vi "_SBR_mes_sp.vi"(6 "SBR_Set":T3={"file_name"="", "HOT/COLD AUTO"=TRUE, "MPI SSB Set"=TRUE, "AUTO時待ち時間（S）"=1.0, "P/V         V/P"=FALSE, "save"=TRUE, "start(GHz)"=4.0, "stop(GHz) "=12.0, "Step(GHz) "=0.1, "P.M.aveg"=10, "PM        SP"=FALSE, "SP_set"={"start(GHz)"=3.5, "stop(GHz) "=12.5, "BW(MHz)"=8.0, "VBW(Hz)"=30.0, "ref(dBm)"=-45.0, "log(dB)"=1.0, "AVEG"=1, "AVEG ON/OFF"=FALSE, "Auto Align ON/OFF"=FALSE, "GPIB"="18", "point"=801}}, 7 "Control":T2={"GPIB_ATT"="28", "6501Dev#"=1, "GPIB_SP"="18", "GPIB_PM"="13", "GPIB_DSA"="11", "GPIB_DMM (TPD)"="23", "MPICOM"="COM5", "mortor設定"=[{"Axis"=0, "ID"=0, "HIspeed"=200.0, "LOspeed"=100.0, "ACCEL(ms)"=100.0, "Sratio"=50.0, "フリーラン\n"=FALSE, "文字列"="DSB HOT/COLD"}, {"Axis"=1, "ID"=0, "HIspeed"=4.0, "LOspeed"=4.0, "ACCEL(ms)"=100.0, "Sratio"=50.0, "フリーラン\n"=TRUE, "文字列"="SubMM Att"}, {"Axis"=0, "ID"=0, "HIspeed"=200.0, "LOspeed"=100.0, "ACCEL(ms)"=100.0, "Sratio"=50.0, "フリーラン\n"=FALSE, "文字列"="MPI Port1"}, {"Axis"=1, "ID"=0, "HIspeed"=200.0, "LOspeed"=100.0, "ACCEL(ms)"=100.0, "Sratio"=50.0, "フリーラン\n"=FALSE, "文字列"="MPI Port2"}], "DATAパス"=path "C:/Documents and Settings/?澤佳?/デスクトップ/data/プロトカ?トリッジ/100811_protC4-5/100814_WCA_P0", "DBパス "=path "Z:/band10/Labview_ALMA/MIX95/test", "comment"="NOLO", "ColdCarts"="003601", "Th"=295.0, "Tc"=77.0, "Set_SIS_volt"=2.096774193548387, "Offset"=0.0, "control"=0, "FreqLO"=796.0, "Set_Mag_Cur"=800.0, "MPI offset(mm)"=22.99, "HOT/COLD"=0} {"HOT/COLD" items=["DSB", "SBR", "GainComp"]; "control" items=["CLOSE LOOP", "OPEN LOOP", "Not Control"]}) -> ()   [LabVIEW 2017]
uses:
  <vilib>/express/express arith-compare/Formula/XNode/ExpressFormulaBlockNode.xnode
panel:
  out "XYグラフ 2":cluster{"データ配列":dbl[], "データ配列":dbl[]}[](graph)=[{"データ配列"=[4.0, 4.1, 4.2, 4.3, 4.4, 4.5, 4.6, 4.7, 4.8, 4.9, 5.0, 5.1, 5.2, 5.3, 5.4, 5.5, 5.6, 5.7, 5.8, 5.9, 6.0, 6.1, 6.2, 6.3, 6.4, 6.5, 6.6, 6.7, 6.8, 6.9, 7.0, 7.1, 7.2, 7.3, 7.4, 7.5, 7.6, 7.7, 7.8, 7.9, 8.0, 8.1, 8.2, 8.3, 8.4, 8.5, 8.6, 8.7, 8.8, 8.9, 9.0, 9.1, 9.2, 9.3, 9.4, 9.5, 9.6, 9.7, 9.8, 9.9, 10.0, 10.1, 10.2, 10.3, 10.4, 10.5, 10.6, 10.7, 10.8, 10.9, 11.0, 11.1, 11.2, 11.3, 11.4, 11.5, 11.6, 11.7, 11.8, 11.9, 12.0], "データ配列"=[0.9249046199806905, 0.7517460823312963, 0.9540395840198505, 0.9269162846964503, 0.8135071464293695, 0.6845118078872291, 0.5940848741555105, 0.6595267429496003, 0.8424905890766325, 0.6848614491447951, 0.7468632569240828, 0.7017022540247116, 0.5009781568393058, 0.5420517670471693, 0.6567512705093524, 0.5260819433781404, 0.3738892851233047, 0.5210577608576411, 0.4868080144723247, 0.3748668646829679, 0.40851305214688144, 0.2837618549546105, 0.31906128888492447, 0.29578752754072546, 0.186091340659989, 0.21398760146405285, 0.10777417863579805, 0.149529503683046, 0.07958880444948759, 0.07954748815261764, 0.1259459192415544, 0.03515471930494699, 0.048843010718681204, 0.03171586659857754, 0.03513774392157607, 0.01818671370440185, -0.01621661399776954, -0.007299958166486085, 0.03223525679436591, 0.02731107388958061, 0.01199917327442536, 0.042416189630546657, 0.003649695010670608, 0.0016649617408312201, -0.05337023868420484, 0.003002871580193121, -0.06506068611910158, -0.049621795287776015, 0.046733111271247955, 0.012088382838128539, -0.038328518852154166, -0.10639347213811458, -0.061303944619701796, -0.09216414898512537, -0.14209487210153343, -0.15469411614691805, 0.022323601941448917, -0.04899532047290484, -0.10942566444854036, -0.14096019154058603, 0.0905989021163112, -0.0391739187880516, -0.026618766005445365, -0.11471481804298753, -0.1521656000206294, -0.02971053894241202, -0.06853941673839113, -0.15295352656935207, -0.18282933440970475, -0.23669712055460096, -0.33420193764281625, 0.14151372779511212, 0.11668493408571631, 0.06016340251879209, 0.00990019059975937, -0.06182303914612333, -0.12488763229092192, 0.2108352941071432, 0.1546641658899227, 0.09675663767559298, 0.0385754646352136]}, {"データ配列"=[4.0, 4.1, 4.2, 4.3, 4.4, 4.5, 4.6, 4.7, 4.8, 4.9, 5.0, 5.1, 5.2, 5.3, 5.4, 5.5, 5.6, 5.7, 5.8, 5.9, 6.0, 6.1, 6.2, 6.3, 6.4, 6.5, 6.6, 6.7, 6.8, 6.9, 7.0, 7.1, 7.2, 7.3, 7.4, 7.5, 7.6, 7.7, 7.8, 7.9, 8.0, 8.1, 8.2, 8.3, 8.4, 8.5, 8.6, 8.7, 8.8, 8.9, 9.0, 9.1, 9.2, 9.3, 9.4, 9.5, 9.6, 9.7, 9.8, 9.9, 10.0, 10.1, 10.2, 10.3, 10.4, 10.5, 10.6, 10.7, 10.8, 10.9, 11.0, 11.1, 11.2, 11.3, 11.4, 11.5, 11.6, 11.7, 11.8, 11.9, 12.0], "データ配列"=[0.8608442548458806, 0.7044947061255087, 0.942586230446133, 0.8493423462533632, 0.7498852904990045, 0.6081560581526015, 0.5430236262647461, 0.6112878364871215, 0.7766440219127979, 0.6149782219119803, 0.6572667110064123, 0.6314153665922547, 0.42698388986216995, 0.42556280195907853, 0.6250719853321322, 0.46430207183002675, 0.33449694284816134, 0.3882474607513784, 0.41506556549956136, 0.3095955000245737, 0.3439051059443347, 0.18240325622893133, 0.28216500097201935, 0.21140353248088684, 0.09413496569057882, 0.17821059451244267, 0.02989001559470223, 0.08828842570711844, 0.050866182648811285, 0.05573387700815249, 0.0663662835217892, 0.0060675597842494156, 0.025335116139840193, -0.04466065840811484, -0.0009333943257959284, -0.05014719752768275, -0.03863850457661142, -0.05952305731929579, -0.037721361400900405, -0.057166062404831075, -0.02916814808995304, -0.012193201434749976, -0.05312032998266237, -0.03611908754398227, -0.1487916724233145, -0.0936345982389959, -0.11305505580370279, -0.1339112513602761, -0.06524335069777229, -0.05628499636478335, -0.11671426437024365, -0.12007755334931655, -0.07430213142730542, -0.1433316372459072, -0.19742493600277894, -0.24364724201221805, -0.08095792610453033, -0.11881261902412663, -0.18295836886949077, -0.1796637370590902, -0.0021771227974171498, -0.026775088377075353, -0.0733922953710137, -0.21148011251519863, -0.21732805814513603, -0.10245993628641197, -0.15420496911591877, -0.19693792604968408, -0.25066612288482537, -0.32217008482607234, -0.39040508822987946, 0.10341354358296367, 0.0815119128548301, -0.0023439054432579094, -0.09006479558012595, -0.1407232856746613, -0.1823207569229413, 0.17679562449456773, 0.08239435268162094, 0.017011997383429706, -0.016509469169492315]}]
  out "XYグラフ 3":cluster{"データ配列":dbl[], "データ配列":dbl[]}[](graph)=[{"データ配列"=[846.0, 845.9, 845.8, 845.7, 845.6, 845.5, 845.4, 845.3, 845.2, 845.1, 845.0, 844.9, 844.8, 844.7, 844.6, 844.5, 844.4, 844.3, 844.2, 844.1, 844.0, 843.9, 843.8, 843.7, 843.6, 843.5, 843.4, 843.3, 843.2, 843.1, 843.0, 842.9, 842.8, 842.7, 842.6, 842.5, 842.4, 842.3, 842.2, 842.1, 842.0, 841.9, 841.8, 841.7, 841.6, 841.5, 841.4, 841.3, 841.2, 841.1, 841.0, 840.9, 840.8, 840.7, 840.6, 840.5, 840.4, 840.3, 840.2, 840.1, 840.0, 839.9, 839.8, 839.7, 839.6, 839.5, 839.4, 839.3, 839.2, 839.1, 839.0, 838.9, 838.8, 838.7, 838.6, 838.5, 838.4, 838.3, 838.2, 838.1, 838.0], "データ配列"=[548.6440300868269, 532.3446978159301, 548.2566145023541, 544.9061292459833, 538.3138371670094, 526.7499707435629, 519.9997703838006, 527.593359910926, 538.6649629641214, 528.8783476971857, 531.9759636549385, 528.4548463210765, 513.5100557424433, 516.344277513952, 524.5874165109195, 514.3547194297134, 503.7653656940615, 515.5843212692465, 511.0783598537313, 507.55375171659057, 505.8555142030906, 497.52972774878066, 501.23367501224743, 498.1244938121795, 489.8630053526426, 493.1999495623687, 486.236254971209, 488.3096964717638, 482.9518498217425, 485.03073723710247, 486.70267213607735, 480.58951323335924, 482.1108023321396, 481.7962553542322, 480.2342668763604, 480.1246358814105, 478.34749024616036, 479.50312619911205, 480.8342642556151, 480.11632993657906, 480.09010262034064, 481.33419008499317, 479.94632437429556, 479.2444411258671, 475.56007043143904, 479.92516925660385, 474.2701582066877, 475.40266728367556, 479.1159951944159, 479.7010196459051, 475.52458759109373, 472.89567054194913, 473.80662563539966, 472.1704784340717, 468.6585989006322, 468.80409014491283, 479.386903232559, 475.6610934283412, 469.07237974406974, 469.8923820760799, 485.7474282618513, 474.9909858241797, 477.7451890508568, 471.7345659278333, 466.80799840032967, 476.31289425549187, 474.0855612238338, 468.51643935953587, 465.4725917144067, 464.39387004779314, 455.68701805229597, 487.4824379927386, 486.6396397044617, 482.6491011961885, 476.185717770886, 473.69367551401047, 469.2462719814977, 490.9878049262109, 488.417091028331, 483.2977332637604, 478.73867571328907]}, {"データ配列"=[854.0, 854.1, 854.2, 854.3, 854.4, 854.5, 854.6, 854.7, 854.8, 854.9, 855.0, 855.1, 855.2, 855.3, 855.4, 855.5, 855.6, 855.7, 855.8, 855.9, 856.0, 856.1, 856.2, 856.3, 856.4, 856.5, 856.6, 856.7, 856.8, 856.9, 857.0, 857.1, 857.2, 857.3, 857.4, 857.5, 857.6, 857.7, 857.8, 857.9, 858.0, 858.1, 858.2, 858.3, 858.4, 858.5, 858.6, 858.7, 858.8, 858.9, 859.0, 859.1, 859.2, 859.3, 859.4, 859.5, 859.6, 859.7, 859.8, 859.9, 860.0, 860.1, 860.2, 860.3, 860.4, 860.5, 860.6, 860.7, 860.8, 860.9, 861.0, 861.1, 861.2, 861.3, 861.4, 861.5, 861.6, 861.7, 861.8, 861.9, 862.0], "データ配列"=[428.63466788231324, 435.4935786985518, 424.9429241146229, 425.381002919813, 433.20647623071613, 438.7104620965752, 443.67374232684676, 442.41046901070797, 430.10206610123777, 440.4868132571015, 435.759630172149, 438.12370344225775, 449.17411817434277, 446.7229210528855, 440.15843962648995, 446.8897154052984, 455.8583559850793, 448.5867165832221, 448.7198763169121, 459.213527054518, 453.52958129721236, 461.1908621778645, 460.27576536783874, 460.2582724546055, 466.0864670209972, 465.7857212585232, 472.4310313017354, 469.17709649506514, 472.78362850317023, 474.8300149659003, 470.5899912757829, 476.0942267925349, 475.8579793140339, 477.7303156869513, 475.74400495243003, 477.79647352046953, 480.42504158528186, 480.43932637294694, 476.7091000205245, 476.62383716173747, 478.55303619667967, 475.9076566852461, 479.478478145908, 479.03123367121594, 482.39234918165187, 479.54022383471187, 482.5907823874182, 481.7505278760315, 473.16388160930836, 478.15362306779105, 480.4224566467349, 486.5333822347131, 481.63681143700416, 483.9492838089557, 486.8070352464491, 488.59582820525645, 476.5343014109415, 481.9312913888416, 483.0061248872076, 487.93423410039685, 474.129463031071, 479.9925386625467, 481.15577320464706, 486.42199876382404, 486.19935785269905, 480.1111428291795, 482.85166491000814, 488.0712289584561, 488.79712182957707, 494.7195539445724, 498.2972613667672, 469.3853698503216, 471.69756792095194, 474.9496602642304, 474.9261101258189, 481.58901751620425, 485.18240521858206, 464.0725253238966, 468.63537032154585, 470.95286464714934, 473.82427991781964]}]
  out "1Dデータ":dbl[](array[numeric])=[12.0, -12.8080699, -13.8899317, -15.3493734, -13.8931044, -15.3471664, 19.85991633178654, 0.0]
  out "XYグラフ":cluster{"データ配列":dbl[], "データ配列":dbl[]}[](graph)
  in  "Tin":T1(ring)=enum."3: C/C"
  in  "OKボタン":bool
  out "wait":dbl=964.9493337
  in  "タブ制御器":enum32{"ページ 1", "ページ 2", "ページ 3"}(tab)
  out "MPI SBR(dB)":dbl=19.65107286127357
  out "MU（mag）":dbl=0.6324558993924078
  out "ML（mag）":dbl=0.006853666405205144
  out "MPIPOS（mm）":dbl=19.85991633178654
  out "データ配列":dbl[][](array[numeric])
  out "SBRAクラスタ":T4={"データ配列"=array801x17[13617 elements], "Points"=801, "Th"=297.0, "Tc"=77.0, "LO(GHz)"=0.0, "Offset(mm)"=0.0, "Pos(mm)"=0.0, "P/V         V/P"=FALSE, "AUTOSAVE"=TRUE, "file_name"="", "パス"=path "", "header+(filename)"="A_"}
  # "Port"
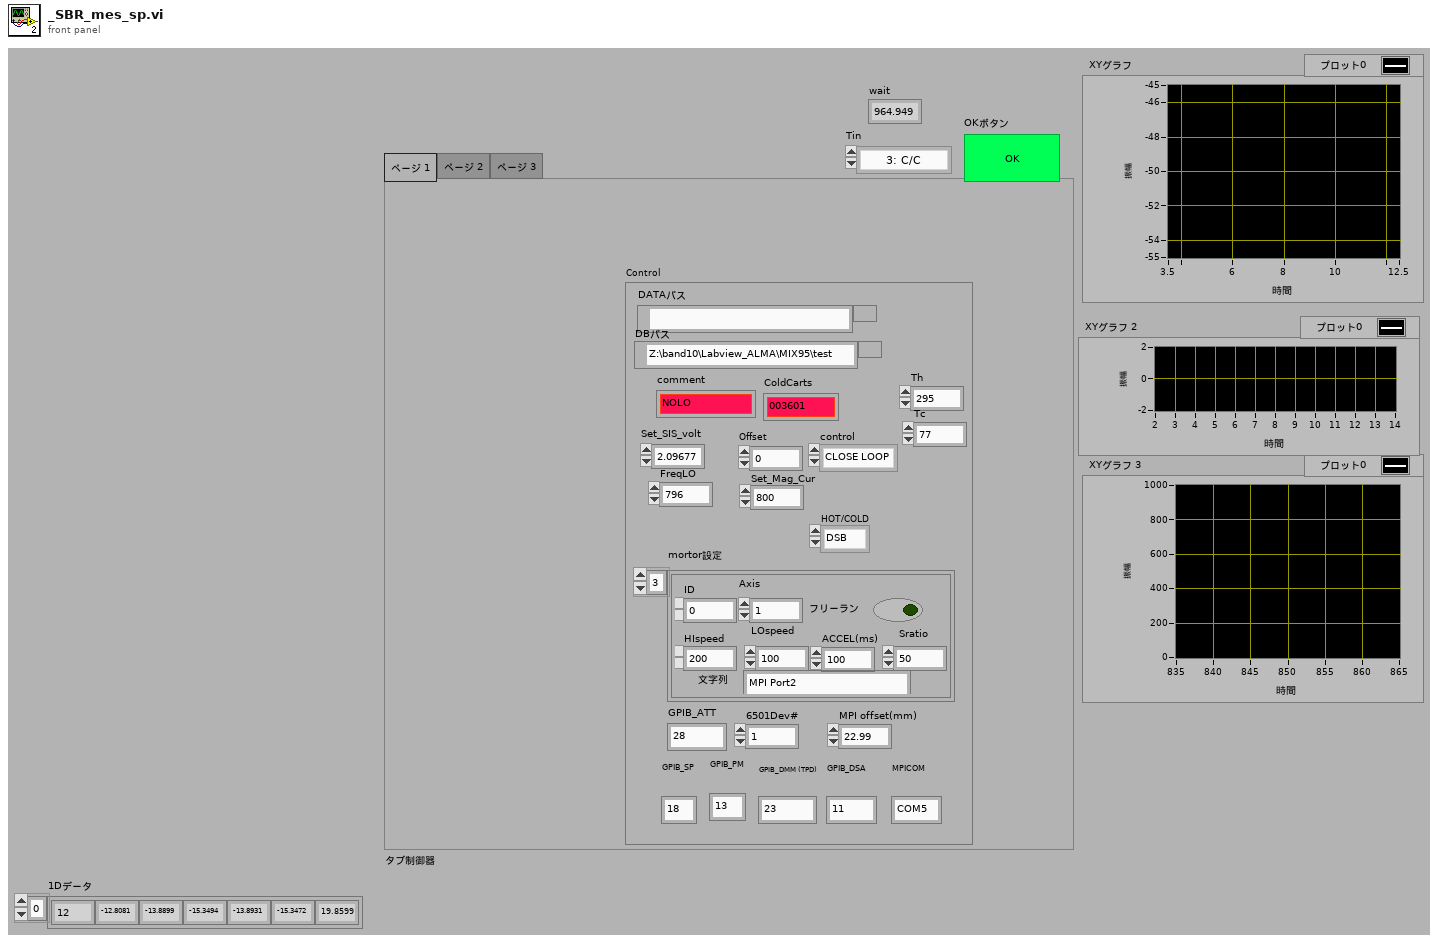
[diagram p1: front panel]
types:
  T1 = enum16{"1: H/H", "2: H/C", "3: C/C", "4: C/H", "5: H/H"}
  T2 = cluster{"GPIB_ATT":string, "6501Dev#":i16, "GPIB_SP":string, "GPIB_PM":string, "GPIB_DSA":string, "GPIB_DMM (TPD)":string, "MPICOM":string, "mortor設定":cluster{"Axis":i16, "ID":i16, "HIspeed":dbl, "LOspeed":dbl, "ACCEL(ms)":dbl, "Sratio":dbl, "フリーラン\n":bool, "文字列":string}[], "DATAパス":path, "DBパス ":path, "comment":string, "ColdCarts":string, "Th":dbl, "Tc":dbl, "Set_SIS_volt":dbl, "Offset":dbl, "control":u16, "FreqLO":dbl, "Set_Mag_Cur":dbl, "MPI offset(mm)":dbl, "HOT/COLD":u16}
  T3 = cluster{"file_name":string, "HOT/COLD AUTO":bool, "MPI SSB Set":bool, "AUTO時待ち時間（S）":dbl, "P/V         V/P":bool, "save":bool, "start(GHz)":dbl, "stop(GHz) ":dbl, "Step(GHz) ":dbl, "P.M.aveg":i32, "PM        SP":bool, "SP_set":cluster{"start(GHz)":dbl, "stop(GHz) ":dbl, "BW(MHz)":dbl, "VBW(Hz)":dbl, "ref(dBm)":dbl, "log(dB)":dbl, "AVEG":i16, "AVEG ON/OFF":bool, "Auto Align ON/OFF":bool, "GPIB":string, "point":i16}}
  T4 = cluster{"データ配列":dbl[][], "Points":i32, "Th":dbl, "Tc":dbl, "LO(GHz)":dbl, "Offset(mm)":dbl, "Pos(mm)":dbl, "P/V         V/P":bool, "AUTOSAVE":bool, "file_name":string, "パス":path, "header+(filename)":string}
  T5 = cluster{"start(GHz)":dbl, "stop(GHz) ":dbl, "BW(MHz)":dbl, "VBW(Hz)":dbl, "ref(dBm)":dbl, "log(dB)":dbl, "AVEG":i16, "AVEG ON/OFF":bool, "Auto Align ON/OFF":bool, "GPIB":string, "point":i16}
  T6 = cluster{"Axis":i16, "ID":i16, "HIspeed":dbl, "LOspeed":dbl, "ACCEL(ms)":dbl, "Sratio":dbl, "フリーラン\n":bool, "文字列":string}[]
  T7 = cluster{"Axis":i16, "ID":i16, "HIspeed":dbl, "LOspeed":dbl, "ACCEL(ms)":dbl, "Sratio":dbl, "フリーラン\n":bool, "文字列":string}
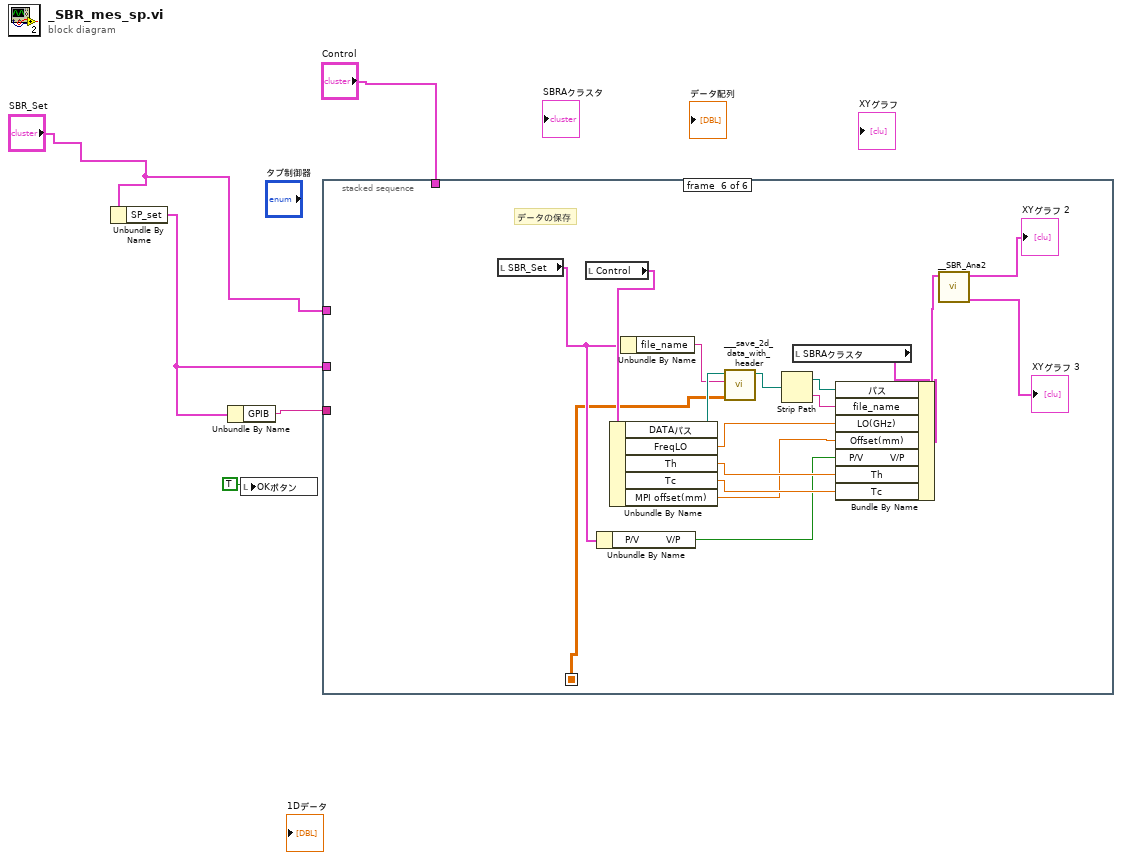
[diagram p0: block diagram]
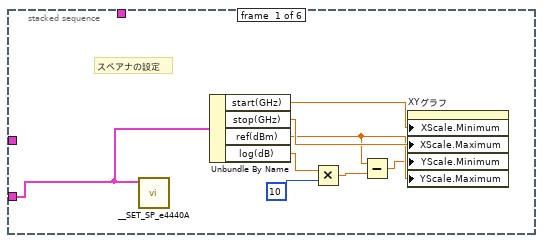
[diagram p2: hidden frame]
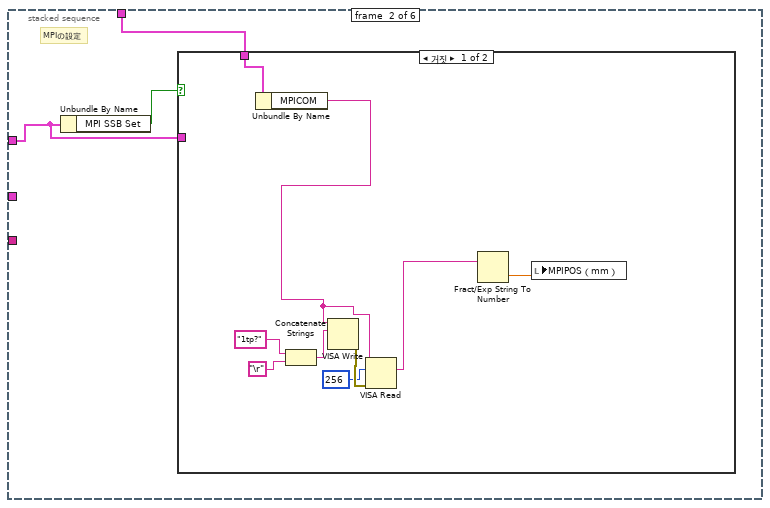
[diagram p3: hidden frame]
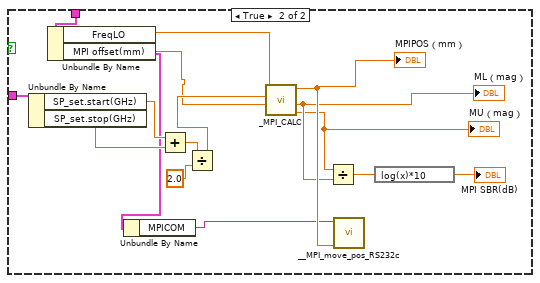
[diagram p4: hidden frame]
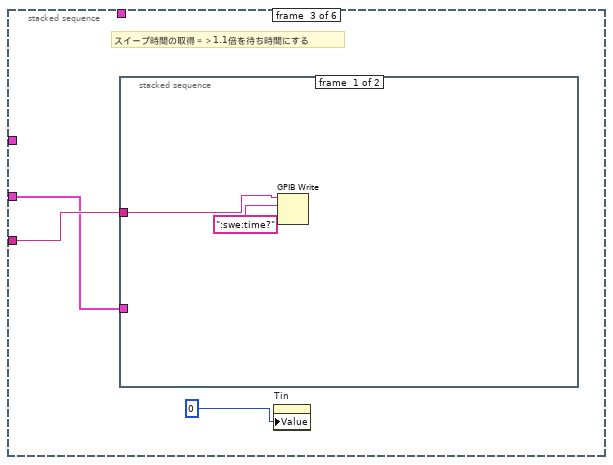
[diagram p5: hidden frame]
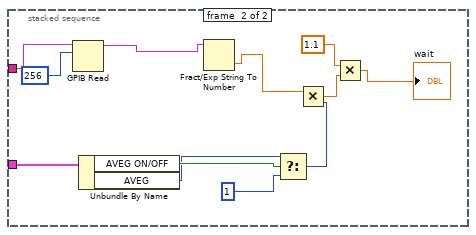
[diagram p6: hidden frame]
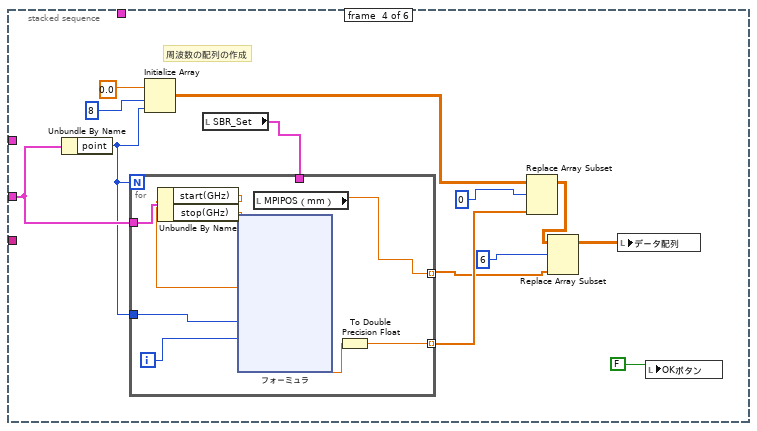
[diagram p7: hidden frame]
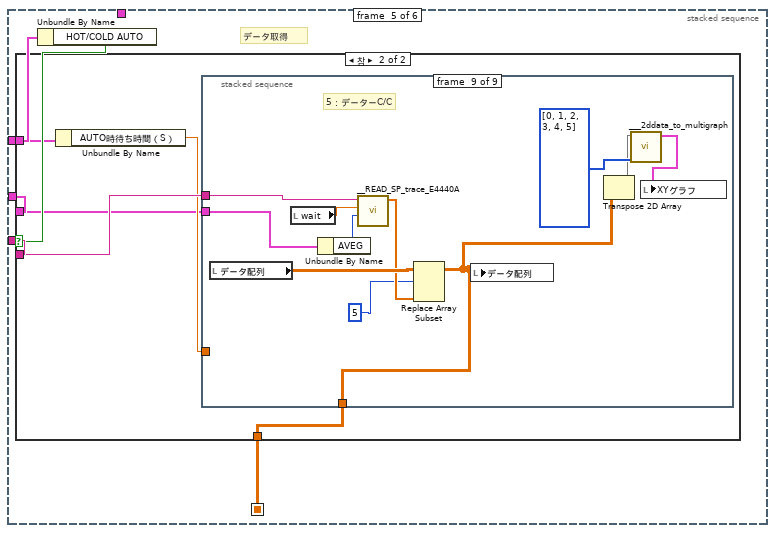
[diagram p8: hidden frame]
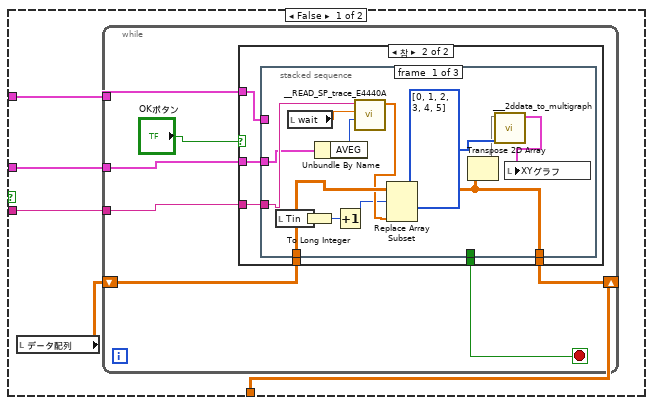
[diagram p9: hidden frame]
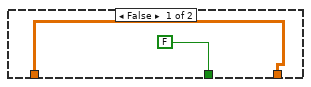
[diagram p10: hidden frame]
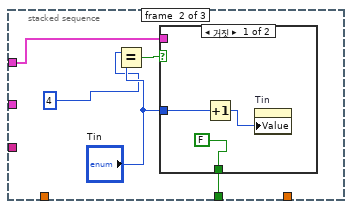
[diagram p11: hidden frame]
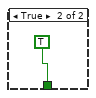
[diagram p12: hidden frame]
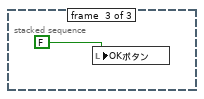
[diagram p13: hidden frame]
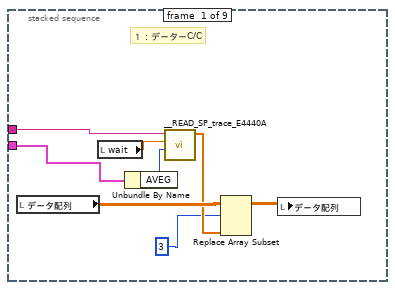
[diagram p14: hidden frame]
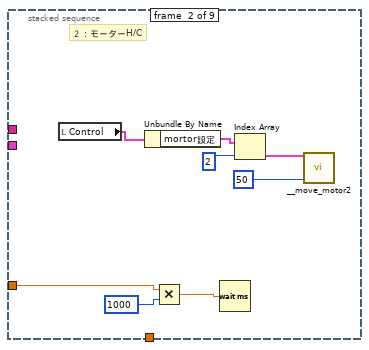
[diagram p15: hidden frame]
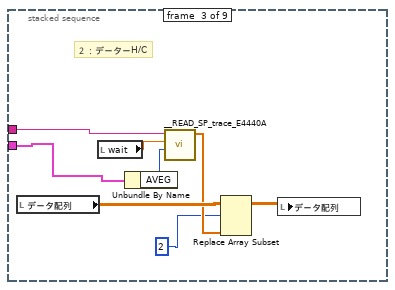
[diagram p16: hidden frame]
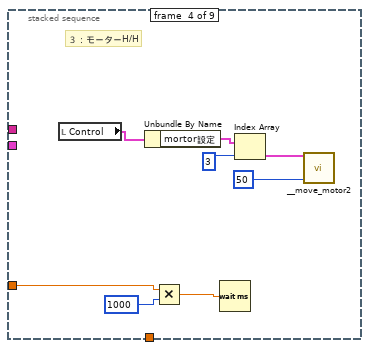
[diagram p17: hidden frame]
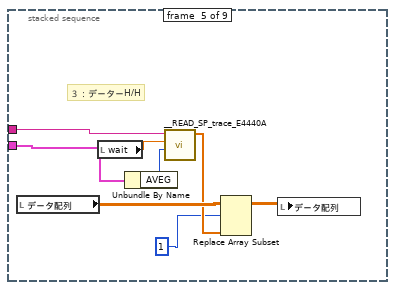
[diagram p18: hidden frame]
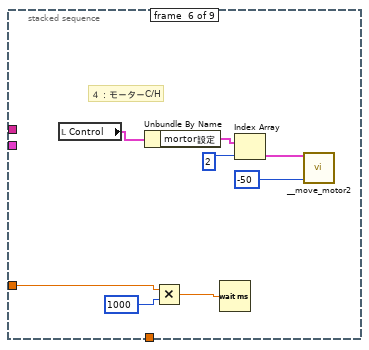
[diagram p19: hidden frame]
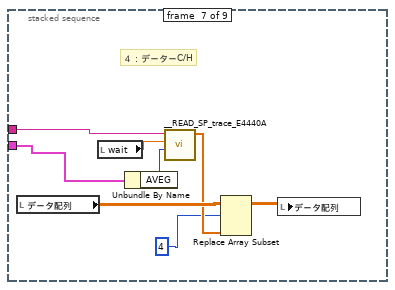
[diagram p20: hidden frame]
diagram:
  n1 = Unbundle By Name("SBR_Set") -> ("SP_set"=w3:T5)
  n2 = Unbundle By Name(w3) -> ("GPIB"=w5:string)
  n3 = local write "OKボタン"(TRUE) -> ()
  n4 = stacked-sequence {
    seq-local: [_ _ _ _ w95 _] -> [_ _ _ _ _ w222]
    tunnel: w3 -> [w13 _ w42 w68 w97 _]
    tunnel: w5 -> [_ _ w43 _ w96 _]
    tunnel: "SBR_Set" -> [_ w15 _ _ w94 _]
    tunnel: "Control" -> [_ w14 _ _ _ _]
    frame #0 {
      # "スペアナの設定"
      n5 = call "__SET_SP_e4440A.vi"("SP"=w13) -> ()  [unwired: 7 in]
      n6 = Unbundle By Name(w13) -> ("start(GHz)"=w12:dbl, "stop(GHz)"=w11:dbl, "ref(dBm)"=w9:dbl, "log(dB)"=w10:dbl)
      n7 = Multiply(x=w10, y=10) -> (x*y=w8:dbl)
      n8 = Subtract(x=w9, y=w8) -> (x-y=w7:dbl)
      n9 = property on="XYグラフ" class="XYGraph (决拜茄)"("XScale.Minimum"=w12, "XScale.Maximum"=w11, "YScale.Minimum"=w7, "YScale.Maximum"=w9) -> ()  [unwired: 2 in, 2 out]
    }
    frame #1 {
      # "MPIの設定"
      n10 = Unbundle By Name(w15) -> ("MPI SSB Set"=w16:bool)
      n11 = case shown="거짓" w16 {
        tunnel: w15 -> [_ w40]
        tunnel: w14 -> [w25 w28]
        frame False {
          n12 = Unbundle By Name(w25) -> ("MPICOM"=w18:string)
          n13 = Concatenate Strings("1tp?", "\r") -> (w20:string)
          n14 = VISA Write(VISA resource name=w18, write buffer=w20) -> (error out=w23:errorcluster)  [unwired: 1 in, 2 out]
          n15 = VISA Read(VISA resource name=w18, byte count=256, error in (no error)=w23) -> (read buffer=w17:string)  [unwired: 3 out]
          n16 = Fract/Exp String To Number(string=w17) -> (number=w24:dbl)  [unwired: 3 in, 1 out]
          n17 = local write "MPIPOS（mm）"(w24) -> ()
        }
        frame True {
          n18 = Unbundle By Name(w40) -> ("SP_set.start(GHz)"=w37:dbl, "SP_set.stop(GHz)"=w36:dbl)
          n19 = Unbundle By Name(w28) -> ("FreqLO"=w38:dbl, "MPI offset(mm)"=w26:dbl)
          n20 = Unbundle By Name(w28) -> ("MPICOM"=w27:string)
          n21 = Add(x=w37, y=w36) -> (x+y=w35:dbl)
          n22 = Divide(x=w35, y=2.0) -> (x/y=w33:dbl)
          n23 = call "_MPI_CALC.vi"("ofset (mm)"=w26, "IF（GHｚ）"=w33, "LO（GHｚ）"=w38) -> ("PU (mag)"=w30:dbl, "PL (lmag)"=w31:dbl, "SSB_pos(mm)"=w32:dbl)  [unwired: 6 in]
          "MU（mag）" <- w30
          "MPIPOS（mm）" <- w32
          "ML（mag）" <- w31
          n24 = Divide(x=w30, y=w31) -> (x/y=w39:dbl)
          n25 = call "__MPI_move_pos_RS232c.vi"("pos"=w32, "VISAリソース名"=w27) -> ()  [unwired: 5 in, 1 out]
          n26 = expression code="log(x)*10"(w39) -> (→"MPI SBR(dB)":dbl)
        }
      }
    }
    frame #2 {
      # "スイープ時間の取得＝＞1.1倍を待ち時間にする"
      n27 = stacked-sequence {
        tunnel: w43 -> [w44 w55]
        tunnel: w42 -> [_ w54]
        frame #0 {
          n28 = GPIB Write(0:w44, 1:":swe:time?") -> ()  [unwired: 3 in, 2 out]
        }
        frame #1 {
          n29 = GPIB Read(0:w55, 1:256) -> (5:w56:string)  [unwired: 3 in, 2 out]
          n30 = Unbundle By Name(w54) -> ("AVEG ON/OFF"=w53:bool, "AVEG"=w52:i16)
          n31 = Fract/Exp String To Number(string=w56) -> (number=w49:dbl)  [unwired: 3 in, 1 out]
          n32 = Select(t=w52, s=w53, f=1) -> (s? t:f=w50:i32)
          n33 = Multiply(x=w49, y=w50) -> (x*y=w47:dbl)
          n34 = Multiply(x=1.1, y=w47) -> (x*y=→"wait":dbl)
        }
      }
      n35 = property on="Tin" class="Enum (决拜茄)"("Value"=0) -> ()  [unwired: 2 in, 2 out]
    }
    frame #3 {
      # "周波数の配列の作成"
      n36 = Unbundle By Name(w68) -> ("point"=w67:i16)
      n37 = Initialize Array(0.0, 8, w67) -> (w65:dbl[][])
      n38 = local read "SBR_Set"() -> (w60:T3)
      n39 = for {
        N: w67 -> [_]
        tunnel: w68 -> [w78]
        tunnel: w67 -> [w76]
        tunnel: [w72] -> w66 mode=indexing
        tunnel: w60 -> [_]
        tunnel: [w71] -> w59 mode=indexing
        i -> [w77]
        n40 = Unbundle By Name(w78) -> ("start(GHz)"=w74:dbl, "stop(GHz)"=w75:dbl)
        n41 = xnode "フォーミュラ"("start"=w74, "stop"=w75, "point"=w76, "num"=w77) -> ("結果"=w73:dbl)  [unwired: 1 in, 1 out]
        n42 = local read "MPIPOS（mm）"() -> (w71:dbl)
        n43 = To Double Precision Float(number=w73) -> (double precision float=w72:dbl)
      }
      n44 = Replace Array Subset(array=w65, new element=w66, index (row)=0) -> (w62:dbl[][])  [unwired: 1 in]
      n45 = Replace Array Subset(array=w62, new element=w59, index (row)=6) -> (w58:dbl[][])  [unwired: 1 in]
      n46 = local write "データ配列"(w58) -> ()
      n47 = local write "OKボタン"(FALSE) -> ()
    }
    frame #4 {
      # "データ取得"
      n48 = Unbundle By Name(w94) -> ("HOT/COLD AUTO"=w93:bool)
      n49 = case shown="참" w93 {
        tunnel: w94 -> [w102 w144]
        tunnel: w97 -> [w101 w142]
        tunnel: w96 -> [w100 w145]
        tunnel: [w99 w141] -> w95
        frame False {
          n50 = local read "データ配列"() -> (w98:dbl[][])
          n51 = while {
            tunnel: w102 -> [w107]
            tunnel: w101 -> [w109]
            tunnel: w100 -> [w108]
            shift-right: [w103] -> w99
            shift-left: w98 -> [w104]
            stop <- w106 stop-if-true
            n52 = case shown="참" "OKボタン" {
              tunnel: w109 -> [_ w117]
              tunnel: w108 -> [_ w116]
              tunnel: w107 -> [_ w115]
              tunnel: [FALSE w114] -> w106
              tunnel: w104 -> [w110 w113]
              tunnel: [w110 w112] -> w103
              frame False {
              }
              frame True {
                n53 = stacked-sequence {
                  tunnel: w117 -> [w125 _ _]
                  tunnel: w116 -> [w128 _ _]
                  tunnel: w115 -> [_ w133 _]
                  tunnel: [_ w134 _] -> w114
                  tunnel: w113 -> [w130 _ _]
                  tunnel: [w121 _ _] -> w112
                  frame #0 {
                    n54 = local read "Tin"() -> (w129:T1)
                    n55 = local read "wait"() -> (w127:dbl)
                    n56 = To Long Integer(number=w129) -> (32bit integer=w119:i32)
                    n57 = Unbundle By Name(w125) -> ("AVEG"=w124:i16)
                    n58 = Increment(x=w119) -> (x+1=w123:i32)
                    n59 = call "__READ_SP_trace_E4440A.vi"("AVG(0-100)"=w124, "wait(s)"=w127, "GPIB"=w128) -> ("data"=w126:dbl[])  [unwired: 3 in, 1 out]
                    n60 = Replace Array Subset(array=w130, new element=w126, index (row)=w123) -> (w121:dbl[][])  [unwired: 1 in]
                    n61 = Transpose 2D Array(2D array=w121) -> (transposed array=w120:dbl[][])
                    n62 = call "___2ddata_to_multigraph.vi"("列"=i32[] [0, 1, 2, 3, 4, 5], "データ配列"=w120) -> ("XYグラフ"=w118:cluster{"データ配列":dbl[], "データ配列":dbl[]}[])  [unwired: 5 in]
                    n63 = local write "XYグラフ"(w118) -> ()
                  }
                  frame #1 {
                    n64 = Equal?(x=4, y="Tin") -> (x = y?=w135:bool)
                    n65 = case shown="거짓" w135 {
                      tunnel: [FALSE TRUE] -> w134
                      tunnel: "Tin" -> [w138 _]
                      tunnel: w133 -> [_ _]
                      frame False {
                        n66 = Increment(x=w138) -> (x+1=w136:T1)
                        n67 = property on="Tin" class="Enum (决拜茄)"("Value"=w136) -> ()  [unwired: 2 in, 2 out]
                      }
                      frame True {
                      }
                    }
                  }
                  frame #2 {
                    n68 = local write "OKボタン"(FALSE) -> ()
                  }
                }
              }
            }
          }
        }
        frame True {
          n69 = Unbundle By Name(w144) -> ("AUTO時待ち時間（S）"=w143:dbl)
          n70 = stacked-sequence {
            tunnel: w145 -> [w151 _ w167 _ w183 _ w199 _ w218]
            tunnel: w143 -> [_ w154 _ w170 _ w186 _ w202 _]
            tunnel: w142 -> [w146 _ w162 _ w178 _ w194 _ w214]
            tunnel: [_ _ _ _ _ _ _ _ w210] -> w141
            frame #0 {
              # "１：データーC/C"
              n71 = local read "データ配列"() -> (w150:dbl[][])
              n72 = local read "wait"() -> (w153:dbl)
              n73 = Unbundle By Name(w146) -> ("AVEG"=w152:i16)
              n74 = call "__READ_SP_trace_E4440A.vi"("AVG(0-100)"=w152, "wait(s)"=w153, "GPIB"=w151) -> ("data"=w149:dbl[])  [unwired: 3 in, 1 out]
              n75 = Replace Array Subset(array=w150, new element=w149, index (row)=3) -> (w147:dbl[][])  [unwired: 1 in]
              n76 = local write "データ配列"(w147) -> ()
            }
            frame #1 {
              # "２：モーターH/C"
              n77 = local read "Control"() -> (w157:T2)
              n78 = Unbundle By Name(w157) -> ("mortor設定"=w156:T6)
              n79 = Multiply(x=w154, y=1000) -> (x*y=w161:dbl)
              n80 = Wait (ms)(milliseconds to wait=w161) -> ()  [unwired: 1 out]
              n81 = Index Array(array=w156, index=2) -> (element=w155:T7)
              n82 = call "__move_motor2.vi"("Moving distance"=50, "motor setup"=w155) -> ()  [unwired: 2 in, 2 out]
            }
            frame #2 {
              # "２：データーH/C"
              n83 = local read "データ配列"() -> (w166:dbl[][])
              n84 = local read "wait"() -> (w169:dbl)
              n85 = Unbundle By Name(w162) -> ("AVEG"=w168:i16)
              n86 = call "__READ_SP_trace_E4440A.vi"("AVG(0-100)"=w168, "wait(s)"=w169, "GPIB"=w167) -> ("data"=w165:dbl[])  [unwired: 3 in, 1 out]
              n87 = Replace Array Subset(array=w166, new element=w165, index (row)=2) -> (w163:dbl[][])  [unwired: 1 in]
              n88 = local write "データ配列"(w163) -> ()
            }
            frame #3 {
              # "３：モーターH/H"
              n89 = local read "Control"() -> (w173:T2)
              n90 = Unbundle By Name(w173) -> ("mortor設定"=w172:T6)
              n91 = Multiply(x=w170, y=1000) -> (x*y=w177:dbl)
              n92 = Wait (ms)(milliseconds to wait=w177) -> ()  [unwired: 1 out]
              n93 = Index Array(array=w172, index=3) -> (element=w171:T7)
              n94 = call "__move_motor2.vi"("Moving distance"=50, "motor setup"=w171) -> ()  [unwired: 2 in, 2 out]
            }
            frame #4 {
              # "３：データーH/H"
              n95 = local read "データ配列"() -> (w182:dbl[][])
              n96 = local read "wait"() -> (w185:dbl)
              n97 = Unbundle By Name(w178) -> ("AVEG"=w184:i16)
              n98 = call "__READ_SP_trace_E4440A.vi"("AVG(0-100)"=w184, "wait(s)"=w185, "GPIB"=w183) -> ("data"=w181:dbl[])  [unwired: 3 in, 1 out]
              n99 = Replace Array Subset(array=w182, new element=w181, index (row)=1) -> (w179:dbl[][])  [unwired: 1 in]
              n100 = local write "データ配列"(w179) -> ()
            }
            frame #5 {
              # "４：モーターC/H"
              n101 = local read "Control"() -> (w189:T2)
              n102 = Unbundle By Name(w189) -> ("mortor設定"=w188:T6)
              n103 = Multiply(x=w186, y=1000) -> (x*y=w193:dbl)
              n104 = Wait (ms)(milliseconds to wait=w193) -> ()  [unwired: 1 out]
              n105 = Index Array(array=w188, index=2) -> (element=w187:T7)
              n106 = call "__move_motor2.vi"("Moving distance"=-50, "motor setup"=w187) -> ()  [unwired: 2 in, 2 out]
            }
            frame #6 {
              # "４：データーC/H"
              n107 = local read "データ配列"() -> (w198:dbl[][])
              n108 = local read "wait"() -> (w201:dbl)
              n109 = Unbundle By Name(w194) -> ("AVEG"=w200:i16)
              n110 = call "__READ_SP_trace_E4440A.vi"("AVG(0-100)"=w200, "wait(s)"=w201, "GPIB"=w199) -> ("data"=w197:dbl[])  [unwired: 3 in, 1 out]
              n111 = Replace Array Subset(array=w198, new element=w197, index (row)=4) -> (w195:dbl[][])  [unwired: 1 in]
              n112 = local write "データ配列"(w195) -> ()
            }
            frame #7 {
              # "５：モーターC/C"
              n113 = local read "Control"() -> (w205:T2)
              n114 = Unbundle By Name(w205) -> ("mortor設定"=w204:T6)
              n115 = Multiply(x=w202, y=1000) -> (x*y=w209:dbl)
              n116 = Wait (ms)(milliseconds to wait=w209) -> ()  [unwired: 1 out]
              n117 = Index Array(array=w204, index=3) -> (element=w203:T7)
              n118 = call "__move_motor2.vi"("Moving distance"=-50, "motor setup"=w203) -> ()  [unwired: 2 in, 2 out]
            }
            frame #8 {
              # "5：データーC/C"
              n119 = local read "データ配列"() -> (w217:dbl[][])
              n120 = local read "wait"() -> (w220:dbl)
              n121 = Unbundle By Name(w214) -> ("AVEG"=w219:i16)
              n122 = call "__READ_SP_trace_E4440A.vi"("AVG(0-100)"=w219, "wait(s)"=w220, "GPIB"=w218) -> ("data"=w216:dbl[])  [unwired: 3 in, 1 out]
              n123 = Replace Array Subset(array=w217, new element=w216, index (row)=5) -> (w210:dbl[][])  [unwired: 1 in]
              n124 = local write "データ配列"(w210) -> ()
              n125 = Transpose 2D Array(2D array=w210) -> (transposed array=w212:dbl[][])
              n126 = call "___2ddata_to_multigraph.vi"("列"=i32[] [0, 1, 2, 3, 4, 5], "データ配列"=w212) -> ("XYグラフ"=w211:cluster{"データ配列":dbl[], "データ配列":dbl[]}[])  [unwired: 5 in]
              n127 = local write "XYグラフ"(w211) -> ()
            }
          }
        }
      }
    }
    frame #5 {
      # "データの保存"
      n128 = local read "SBR_Set"() -> (w223:T3)
      n129 = local read "Control"() -> (w226:T2)
      n130 = Unbundle By Name(w223) -> ("P/V         V/P"=w235:bool)
      n131 = Unbundle By Name(w226) -> ("DATAパス"=w227:path, "FreqLO"=w234:dbl, "Th"=w236:dbl, "Tc"=w237:dbl, "MPI offset(mm)"=w221:dbl)
      n132 = Unbundle By Name(w223) -> ("file_name"=w224:string)
      n133 = call "___save_2d_data_with_header.vi"("配列"=w222, "file_name"=w224, "パス"=w227) -> ("出力パス"=w225:path)  [unwired: 8 in]
      n134 = Strip Path(path=w225) -> (stripped path=w229:path, name=w230:string)
      n135 = local read "SBRAクラスタ"() -> (w228:T4)
      n136 = Bundle By Name(cluster=w228, "パス"=w229, "file_name"=w230, "LO(GHz)"=w234, "Offset(mm)"=w221, "P/V         V/P"=w235, "Th"=w236, "Tc"=w237) -> (w231:T4)
      n137 = call "__SBR_Ana2.vi"("SBRAクラスタ"=w231) -> ("XYグラフ 6"=→"XYグラフ 3":cluster{"データ配列":dbl[], "データ配列":dbl[]}[], "XYグラフ 5"=→"XYグラフ 2":cluster{"データ配列":dbl[], "データ配列":dbl[]}[])  [unwired: 6 in, 1 out]
    }
  }
